vi "Up_Down_Subvi.vi"(9 "Up/Down":enum16{"up", "down"}(ring), 10 "multiplicator":enum16{"1", "10", "100", "1000", "10000"}(ring), 11 "Ref_Totol Number":refnum<vi>) -> (3 "Totol Number":i32)   [LabVIEW 2013]
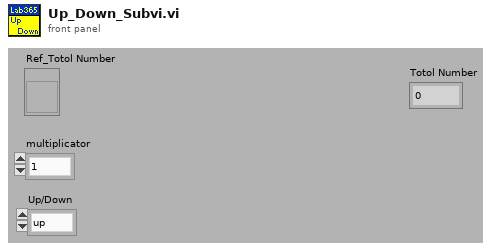
[diagram p1: front panel]
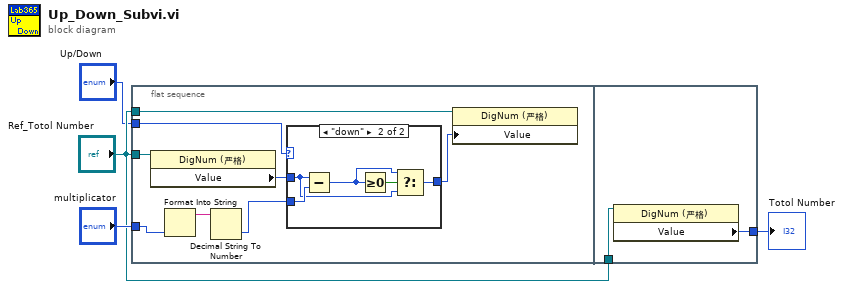
[diagram p0: block diagram]
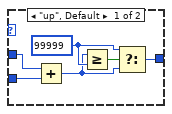
[diagram p2: hidden frame]
diagram:
  n1 = flat-sequence {
    tunnel: "multiplicator" -> [w7]
    tunnel: "Ref_Totol Number" -> [w10]
    tunnel: "Ref_Totol Number" -> [w9]
    tunnel: "Up/Down" -> [w8]
    tunnel: "Ref_Totol Number" -> [w25]
    tunnel: [w24] -> w2
    frame #0 {
      n2 = property class="DigNum (严格)"(reference=w10) -> ("Value"=w12:i32)  [unwired: 1 in, 2 out]
      n3 = Format Into String(w7) -> (resulting string=w6:string)  [unwired: 3 in, 1 out]
      n4 = Decimal String To Number(string=w6) -> (number=w5:i32)  [unwired: 3 out]
      n5 = case shown="\"down\"" w8 {
        tunnel: w12 -> [w18 w19]
        tunnel: [w14 w21] -> w11
        tunnel: w5 -> [w13 w23]
        frame "up", Default {
          w16 = 99999 ("y")
          n6 = Add ("加")(x=w18, y=w13) -> (x+y=w15:i32)
          n7 = Greater Or Equal?(x=w15, y=w16) -> (x >= y?=w17:bool)
          n8 = Select(t=w16, s=w17, f=w15) -> (s? t:f=w14:i32)
        }
        frame "down" {
          n9 = Subtract(x=w19, y=w23) -> (x-y=w20:i32)
          n10 = Greater Or Equal To 0?(x=w20) -> (x >= 0?=w22:bool)
          n11 = Select(t=w20, s=w22, f=w19) -> (s? t:f=w21:i32)
        }
      }
      n12 = property class="DigNum (严格)"(reference=w9, "Value"=w11) -> ()  [unwired: 1 in, 2 out]
    }
    frame #1 {
      n13 = property class="DigNum (严格)"(reference=w25) -> ("Value"=w24:i32)  [unwired: 1 in, 2 out]
    }
  }
  "Totol Number" <- w2
